vi "SS Class Dynamic VI Panel Reference.vi"(10 "Data":variant, 11 "Device Name":string) -> ()   [LabVIEW 2024, in "Subsystem Class.lvclass"]
uses:
  Subsystem Class.lvclass
panel:
  # "This VI provides the template for a dynamic VI that will\nbe implemented by each subsystem."
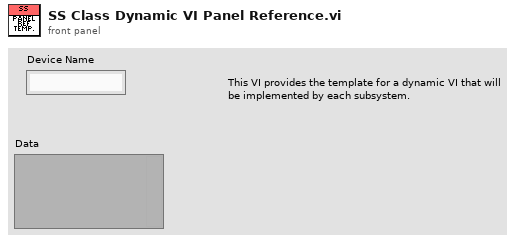
[diagram p1: front panel]
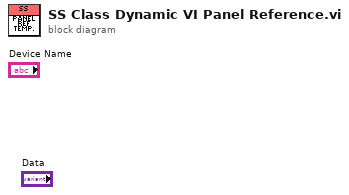
[diagram p0: block diagram]
diagram:
